vi "Launch State Tracker.vi"(11 "RDS Root Actor in":refnum<class "RDS Root Actor.lvclass">) -> (3 "RDS Root Actor out":refnum<class "RDS Root Actor.lvclass">)   [LabVIEW 2015, in "RDS Root Actor.lvlib" / "RDS Root Actor.lvclass"]
uses:
  RDS Root Actor.lvclass
  RDS State Tracker/RDS State Tracker/RDS State Tracker.lvclass
  RDS State Tracker/RDS State Tracker/RDS State Tracker.lvclass/RDS State Tracker.ctl
  RDS Parent Actor/RDS Parent Actor/RDS Parent Actor.lvclass/RDS Parent Actor.ctl
  RDS Parent Actor/RDS Parent Actor/RDS Parent Actor.lvclass
  Libraries/Configuration Library/RDS Configuration Library.lvlib
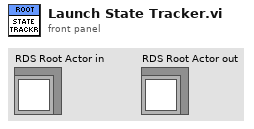
[diagram p1: front panel]
types:
  T1 = typedef "RDS Configuration Library.lvlib/RDS Configuration.ctl" = cluster{"State Update Rate (Hz)":dbl, "Helm Rate (Hz)":dbl, "Helm Gains":T2, "Limiter":dbl, "Mission Controller Settings":T3, "Mag Dev":dbl}
  T2 = typedef "RDS Child Messages.lvlib/PID Gains Control.ctl" = cluster{"P (Kc)":sgl, "I (Ti)":sgl, "D (Td)":sgl}
  T3 = typedef "RDS Mission Controller Actor.lvlib/Mission Controller Settings.ctl" = cluster{"Waypoint Radius (m)":dbl}
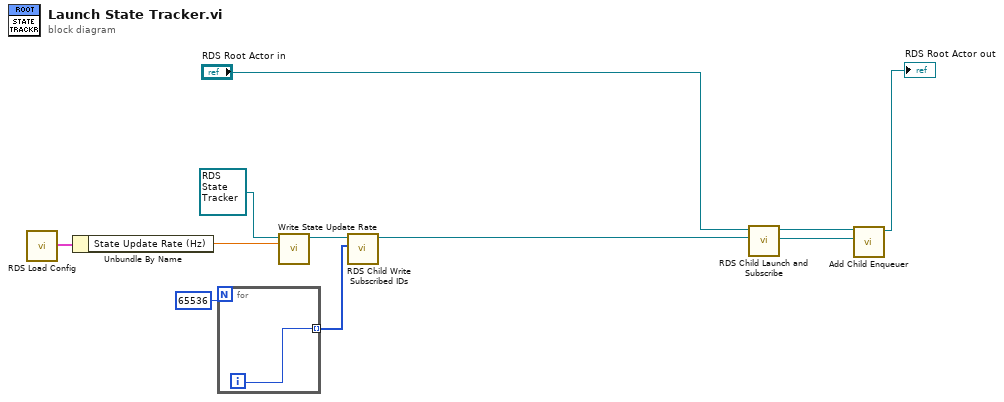
[diagram p0: block diagram]
diagram:
  n1 = call "RDS Load Config.vi"() -> ("RDS Config"=w2:T1)  [unwired: 11 in]
  n2 = Unbundle By Name(w2) -> ("State Update Rate (Hz)"=w1:dbl)
  n3 = for {
    N: 65536 -> [_]
    tunnel: [w12] -> w8 mode=indexing
    i -> [w12]
  }
  n4 = call "Write State Update Rate.vi"("State Update Rate"=w1, "RDS State Tracker in"=refnum<class "RDS State Tracker.lvclass"> refnum ("RDS State Tracker.lvlib:RDS State Tracker.lvclass")) -> ("RDS State Tracker out"=w3:refnum<class "RDS State Tracker.lvclass">)  [unwired: 8 in, 1 out]
  n5 = call "RDS Child Write Subscribed IDs.vi"("Subscribed IDs"=w8, "RDS Parent Actor in"=w3) -> ("RDS Parent Actor out"=w7:refnum<class "RDS State Tracker.lvclass">)  [unwired: 8 in, 1 out]
  n6 = call "RDS Child Launch and Subscribe.vi"("RDS Child in"=w7, "Caller Actor in"="RDS Root Actor in") -> ("Nested Actor's Enqueuer"=w10:refnum<class "Message Enqueuer.lvclass">, "Caller Actor Out"=w9:refnum<class "RDS Root Actor.lvclass">)  [unwired: 7 in, 1 out]
  n7 = call "Add Child Enqueuer.vi"("Nested Actor's Enqueuer"=w10, "RDS Root Actor in"=w9) -> ("RDS Root Actor out"=→"RDS Root Actor out":refnum<class "RDS Root Actor.lvclass">)  [unwired: 8 in, 1 out]
